vi "Signal_Generator.vi"() -> ()   [LabVIEW 2019]
panel:
  out "x+y":dbl
  out "Arbitrary Signal":waveform(dbl)(graph)
  in  "stop":bool
  in  "milliseconds to wait":u32=100
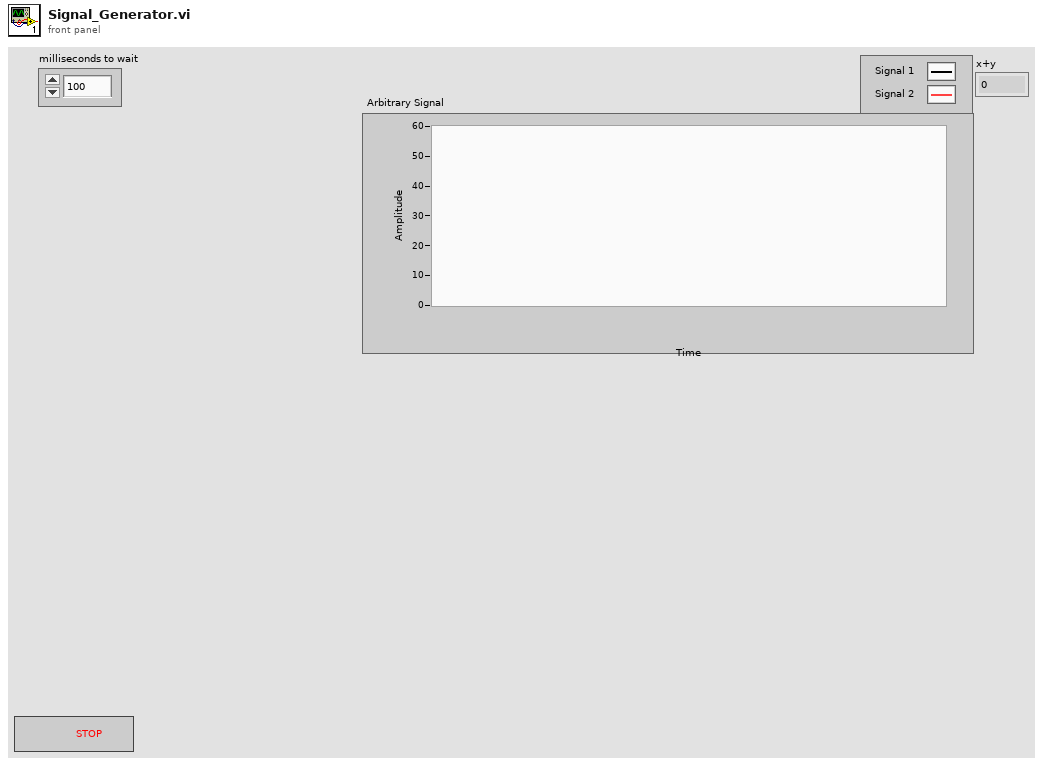
[diagram p1: front panel]
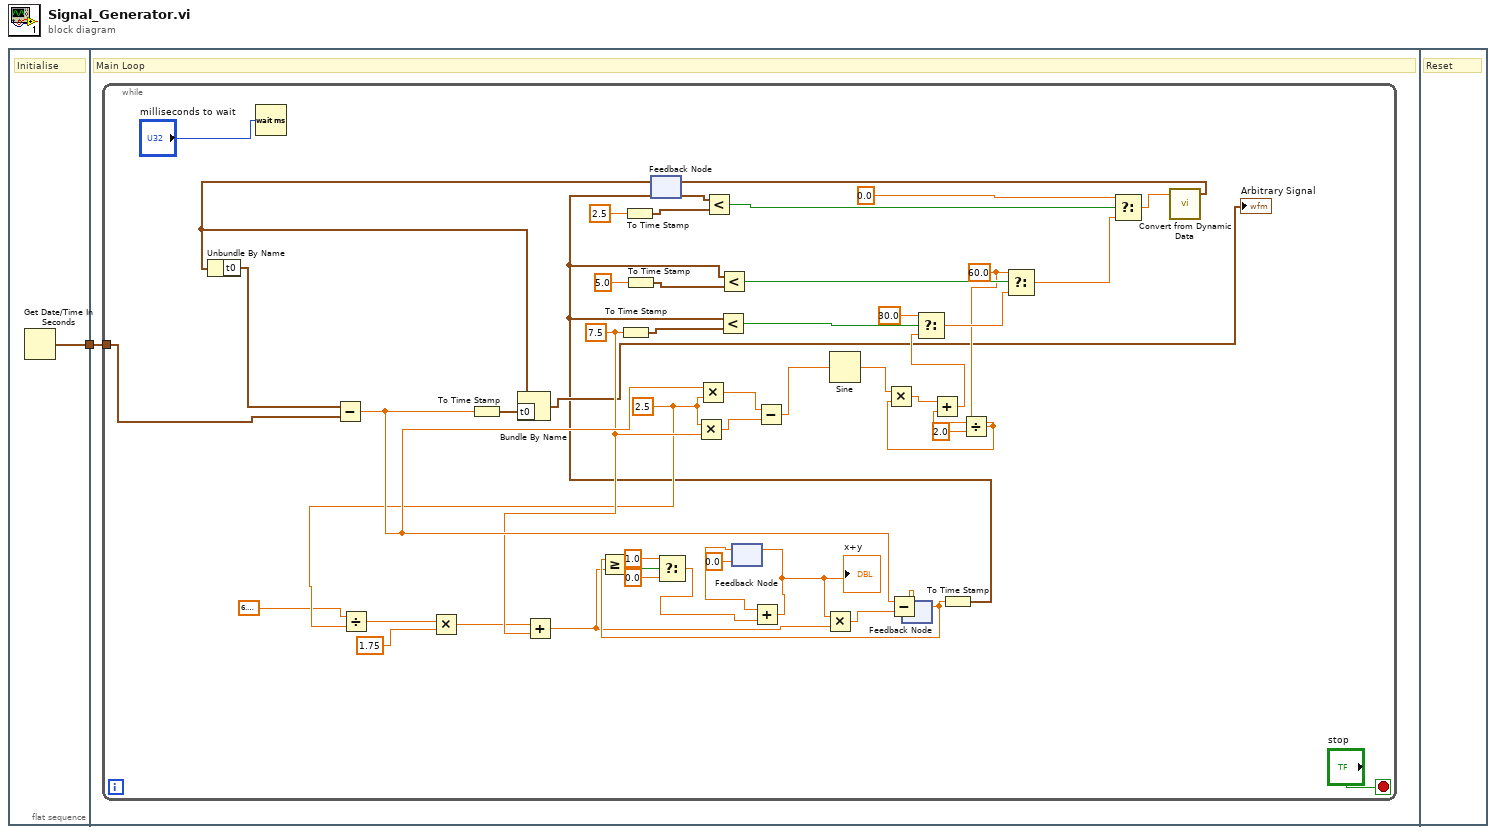
[diagram p0: block diagram]
diagram:
  n1 = flat-sequence {
    tunnel: [w2] -> w1
    tunnel: w1 -> [w3]
    frame #0 {
      # "Initialise"
      n2 = Get Date/Time In Seconds() -> (seconds since 1Jan1904=w2:timestamp)
    }
    frame #1 {
      # "Main Loop"
      n3 = while {
        tunnel: w3 -> [w41]
        stop <- "stop" stop-if-true
        w11 = 2.5 ("y")
        w33 = 60.0 ("t")
        w14 = 7.5 ("number")
        n4 = Wait (ms)(milliseconds to wait="milliseconds to wait") -> ()  [unwired: 1 out]
        n5 = Divide(x=6.283185307179586, y=w11) -> (x/y=w10:dbl)
        n6 = Multiply(x=w10, y=1.75) -> (x*y=w12:dbl)
        n7 = Add(x=w12, y=w14) -> (x+y=w15:dbl)
        n8 = To Time Stamp(1:w14) -> (0:w42:timestamp)
        n9 = To Time Stamp(1:2.5 ("number")) -> (0:w46:timestamp)
        n10 = To Time Stamp(1:5.0 ("number")) -> (0:w43:timestamp)
        n11 = feedback #1() -> (w4:waveform(dbl))  [unwired: 1 in]
        n12 = Unbundle By Name ("Get Waveform Components")(w4) -> ("t0"=w6:timestamp)
        n13 = Subtract(x=w6, y=w41) -> (x-y=w18:dbl)
        n14 = To Time Stamp(1:w18) -> (0:w50:timestamp)
        n15 = Bundle By Name ("Build Waveform")(cluster=w4, "t0"=w50) -> (→"Arbitrary Signal":waveform(dbl))
        n16 = Multiply(x=w11, y=w14) -> (x*y=w29:dbl)
        n17 = Multiply(x=w18, y=w11) -> (x*y=w28:dbl)
        n18 = feedback #2(0.0) -> (w19:dbl)
        n19 = Subtract(x=w28, y=w29) -> (x-y=w30:dbl)
        n20 = Sine(x=w30) -> (sin(x)=w36:dbl)
        n21 = feedback #3() -> (w16:dbl)  [unwired: 1 in]
        n22 = Greater Or Equal?(x=w16, y=w15) -> (x >= y?=w26:bool)
        n23 = Select(t=1.0, s=w26, f=0.0) -> (s? t:f=w20:dbl)
        n24 = Add(x=w19, y=w20) -> (x+y=w21:dbl)
        "x+y" <- w21
        n25 = feedback-in #2(w21) -> ()
        n26 = Multiply(x=w21, y=w15) -> (x*y=w24:dbl)
        n27 = Subtract(x=w18, y=w24) -> (x-y=w17:dbl)
        n28 = feedback-in #3(w17) -> ()
        n29 = To Time Stamp(1:w16) -> (0:w7:timestamp)
        n30 = Less?(x=w7, y=w46) -> (x < y?=w49:bool)
        n31 = Less?(x=w7, y=w42) -> (x < y?=w47:bool)
        n32 = Less?(x=w7, y=w43) -> (x < y?=w48:bool)
        n33 = Divide(x=w33, y=2.0) -> (x/y=w31:dbl)
        n34 = Multiply(x=w36, y=w31) -> (x*y=w35:dbl)
        n35 = Add(x=w35, y=w31) -> (x+y=w34:dbl)
        n36 = Select(t=30.0, s=w47, f=w34) -> (s? t:f=w38:dbl)
        n37 = Select(t=w33, s=w48, f=w38) -> (s? t:f=w39:dbl)
        n38 = Select(t=0.0, s=w49, f=w39) -> (s? t:f=w27:dbl)
        n39 = call "Convert from Dynamic Data"("Dynamic Data Type"=w27) -> ("Waveform"=w5:waveform(dbl))  [unwired: 3 in]
        n40 = feedback-in #1(w5) -> ()
      }
    }
    frame #2 {
      # "Reset"
    }
  }
